vi "Probability Array.vi"(7 "QuWire in":refnum<class "QuWire.lvclass">) -> (4 "Porababilities":dbl[](array[numeric]), 15 "Qubits n":i32)   [LabVIEW 2020]
uses:
  QuSim/QuWire/QuWire.lvclass
panel:
  out "Basis States and Probabilities":cluster{"State":i32, "Probability":dbl}[](array[cluster]) {"Probability" format="%#.6f"; "State" format="%07b"}
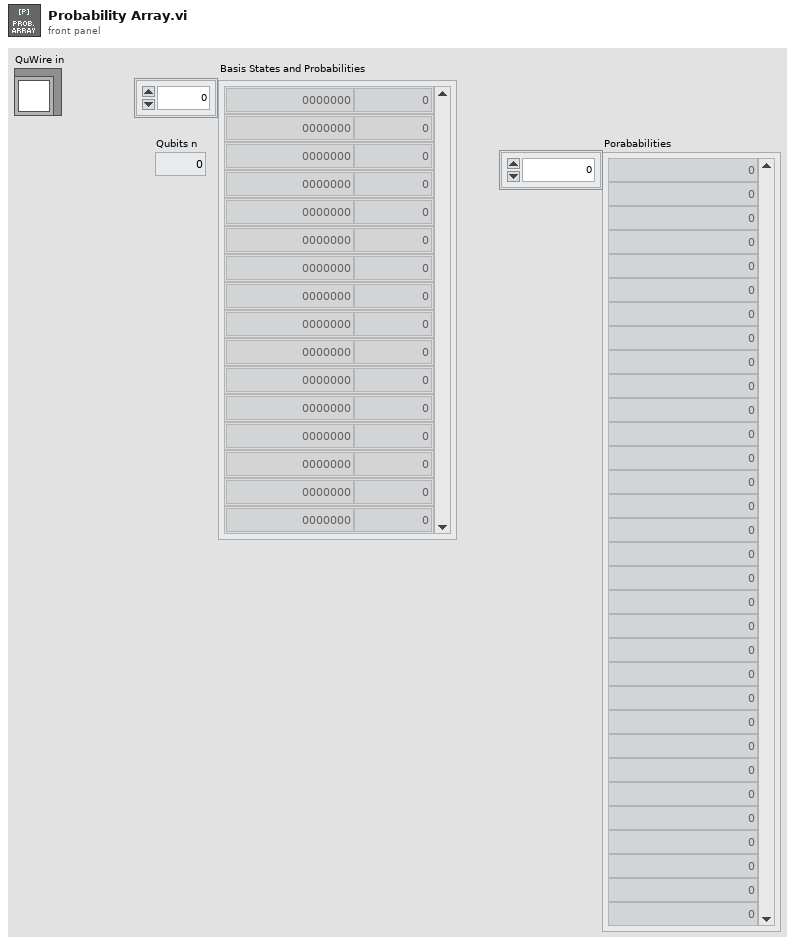
[diagram p1: front panel]
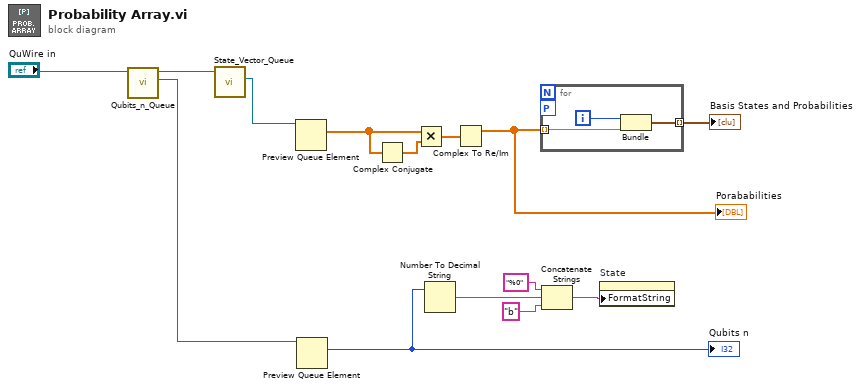
[diagram p0: block diagram]
diagram:
  n1 = call "Qubits_n_Queue.vi"("QuWire in"="QuWire in") -> ("Qubit n"=w8:refnum<queue>, "QuWire out"=w10:refnum<class "QuWire.lvclass">)  [unwired: 8 in, 1 out]
  n2 = call "State_Vector_Queue.vi"("QuWire in"=w10) -> ("State Vector Queue"=w14:refnum<queue>)  [unwired: 8 in, 2 out]
  n3 = Preview Queue Element(queue=w14) -> (element=w12:cdb[])  [unwired: 2 in, 3 out]
  n4 = Preview Queue Element(queue=w8) -> (element=w3:i32)  [unwired: 2 in, 3 out]
  "Qubits n" <- w3
  n5 = Complex Conjugate(1:w12) -> (0:w13:cdb[])
  n6 = Multiply(x=w12, y=w13) -> (x*y=w11:cdb[])
  n7 = Number To Decimal String(number=w3) -> (decimal integer string=w4:string)  [unwired: 1 in]
  n8 = Complex To Re/Im(x + iy=w11) -> (x=w1:dbl[])  [unwired: 1 out]
  "Porababilities" <- w1
  n9 = for {
    tunnel: w1 -> [w16] mode=indexing
    tunnel: [w15] -> w7 mode=indexing
    workers-P: _ -> [_]
    i -> [w17]
    n10 = Bundle(w17, "Complex Matrix Element"=w16) -> (w15:cluster{i32, "Complex Matrix Element":dbl})  [unwired: 1 in]
  }
  "Basis States and Probabilities" <- w7
  n11 = Concatenate Strings("%0" ("string"), w4, "b" ("string")) -> (w2:string)
  n12 = property on="State" class="DigNum (strict)"("FormatString"=w2) -> ()  [unwired: 2 in, 2 out]
